vi "Three singles.vi"(11 "BrickReference in":T1) -> (3 "BrickReference out":T1)   [LabVIEW 2016]
uses:
  <vilib>/NXT/Subs/LVHSConnector.ctl
  <vilib>/NXT/LegoClasses/BrickReference/BrickReference.lvclass
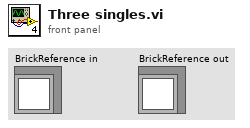
[diagram p1: front panel]
types:
  T1 = typedef "LVHSConnector.ctl" = refnum<class "BrickReference.lvclass">
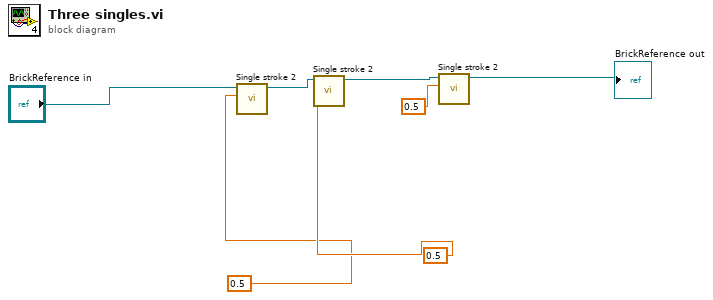
[diagram p0: block diagram]
diagram:
  n1 = call "Single stroke 2.vi"("Numeric"=0.5, "BrickReference in"="BrickReference in") -> ("BrickReference out"=w3:T1)  [unwired: 9 in]
  n2 = call "Single stroke 2.vi"("Numeric"=0.5, "BrickReference in"=w3) -> ("BrickReference out"=w5:T1)  [unwired: 9 in]
  n3 = call "Single stroke 2.vi"("Numeric"=0.5, "BrickReference in"=w5) -> ("BrickReference out"=→"BrickReference out":T1)  [unwired: 9 in]
